vi "ATSh_StartCapture.vi"(11 "Handle":u32) -> (0 "Return Code":u32, 3 "Handle_Out":u32)   [LabVIEW 2015]
doc: "_____AlazarTech, Scope_____\n\nArm the device to initiate an acquisition.\nHandle input."
uses:
  ATSApi.dll
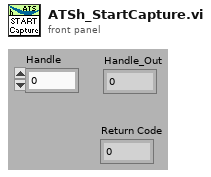
[diagram p1: front panel]
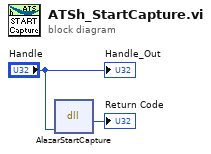
[diagram p0: block diagram]
diagram:
  n1 = dll-call lib="C:/IntensityOCT/trunk/ATSApi.dll" fn="AlazarStartCapture"("h"="Handle") -> (→"Return Code":u32)  [unwired: 4 in, 2 out]
  "Handle_Out" <- "Handle"
